vi "Read Line.vi"(1 "Configuration Bits":T1 items=["Ch 0 SE"=8, "Ch 1 SE"=9, "Ch 2 SE"=10, "Ch 3 SE"=11, "Ch 4 SE"=12, "Ch 5 SE"=13, "Ch 6 SE"=14, "Ch 7 SE"=15, "Diff 0+ 1-"=0, "Diff 1+ 0-"=1, "Diff 2+ 3-"=2, "Diff 3+ 2-"=3, "Diff 4+ 5-"=4, "Diff 5+ 4-"=5, "Diff 6+ 7-"=6, "Diff 7+ 6-"=7], 2 "ADC CS line":refnum<k21>="AI_CS1") -> (0 "number":u16)   [LabVIEW 2018, in "MCP3008.lvlib"]
uses:
  MCP3008.lvlib
  Configuration Bits.ctl
  <vilib>/rvi/eio/common/nirviEmuTemplateMethod_errors.vi
  <vilib>/eio/EIONode/EIONode.xnode
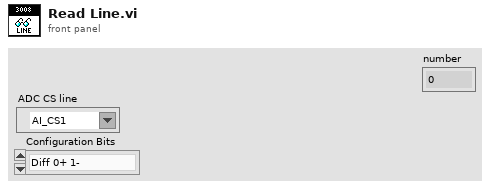
[diagram p1: front panel]
types:
  T1 = typedef "MCP3008.lvlib/Configuration Bits.ctl" = u8
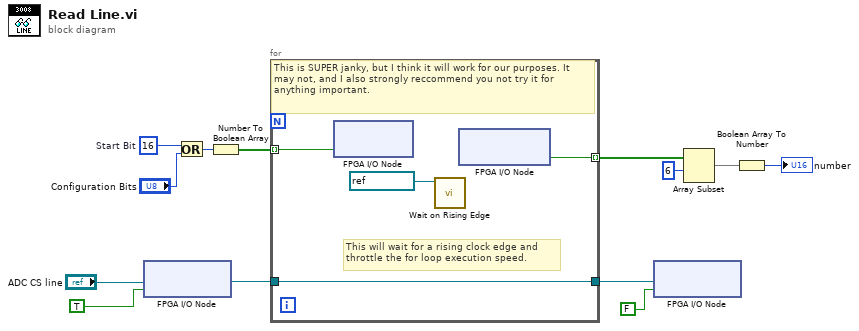
[diagram p0: block diagram]
diagram:
  w8 = u16 16  # Start Bit
  n1 = xnode "FPGA I/O Node"("I/O Item"=TRUE, "FPGA I/O In"="ADC CS line") -> ("FPGA I/O Out"=w2:refnum<k21>)
  n2 = Or(x=w8, y="Configuration Bits") -> (x .or. y?=w9:u16)
  n3 = Number To Boolean Array(number=w9) -> (Boolean array=w10:bool[])
  n4 = for {
    tunnel: w10 -> [w16] mode=indexing
    tunnel: [w17] -> w7 mode=indexing
    tunnel: [w14] -> w1
    tunnel: w2 -> [w14]
    # "This will wait for a rising clock edge and \nthrottle the for loop execution speed."
    # "This is SUPER janky, but I think it will work for our purposes. It may not, and I also strongly reccommend you not try it for anything important."
    n5 = xnode "FPGA I/O Node"("AI_DIN"=w16) -> ()  [unwired: 1 in, 1 out]
    n6 = call "Wait on Rising Edge.vi"("Refnum in"=refnum<k21> "AI_CLK" ("FPGA I/O In")) -> ()  [unwired: 11 in]
    n7 = xnode "FPGA I/O Node"() -> ("AI_DOUT"=w17:bool)  [unwired: 1 in, 1 out]
  }
  n8 = xnode "FPGA I/O Node"("I/O Item"=FALSE, "FPGA I/O In"=w1) -> ()  [unwired: 1 out]
  n9 = Array Subset(array=w7, index=6) -> (w5:bool[])  [unwired: 1 in]
  n10 = Boolean Array To Number(Boolean array=w5) -> (number=→"number":u16)
